vi "ExternalSensorsDataString.vi"(0 "External Sensors In":dbl[](array[numeric])) -> (1 "concatenated string":string)   [LabVIEW 2009]
uses:
  lib/Global Data/Names/Name Actions.ctl
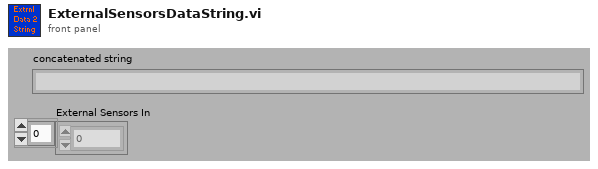
[diagram p1: front panel]
types:
  T1 = typedef "Name Actions.ctl" = enum16{"Init", "Get Names", "Get Index"}
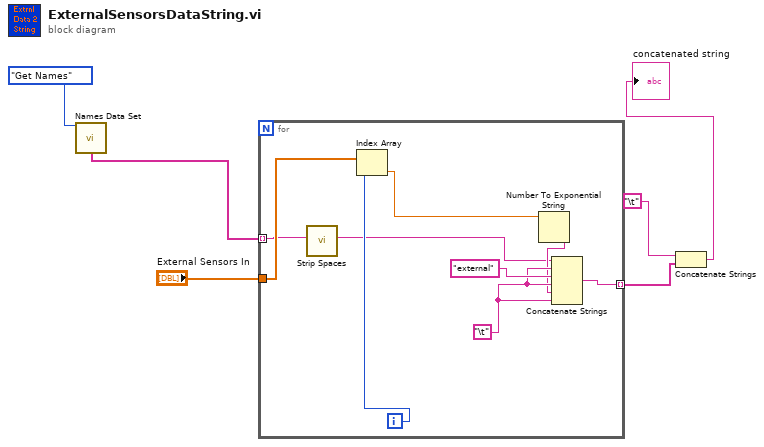
[diagram p0: block diagram]
diagram:
  n1 = call "Names Data Set.vi"("Name Actions"=Name_Actions."Get Names") -> ("External Sensor Names"=w1:string[])  [unwired: 1 in, 13 out]
  n2 = for {
    tunnel: [w15] -> w6 mode=indexing
    tunnel: w1 -> [w8] mode=indexing
    tunnel: "External Sensors In" -> [w11]
    i -> [w10]
    w13 = "\t"
    n3 = call "Strip Spaces.vi"("input string"=w8) -> ("result string"=w7:string)  [unwired: 10 out]
    n4 = Index Array(array=w11, index=w10) -> (element=w9:dbl)
    n5 = Number To Exponential String(number=w9) -> (E-format string=w12:string)  [unwired: 3 out]
    n6 = Concatenate Strings(w7, w13, "external", w13, w12, w13) -> (w15:string)
  }
  n7 = Concatenate Strings("\t", w6) -> (→"concatenated string":string)
